vi "Toobar UI.vi"() -> ()   [LabVIEW 2016]
uses:
  System.Windows.Forms
  ToolKit/Toolbar/net/SubVIs/Pravite/ToolStrip.lvclass
  ToolKit/Toolbar/net/SubVIs/TBA_NET_Item.ctl
  <vilib>/Utility/error.llb/DialogType.ctl
  Architecture/Queue Management/ARC_Queue Create_Single.vi
  Architecture/Queue Management/ARC_Queue Remove Element.vi
  Architecture/Queue Management/ARC_Queue Insert Element.vi
  Architecture/Queue Management/ARC_Queue Destroy_Single.vi
  Architecture/Queue Management/ARC_Queue Valid.vi
panel:
  in  "ToolStrip":refnum<k24>(container)
  in  "Parameter":cluster{"Q_Local":string, "变体":variant}
  in  "TempVariable":T2 {"TBAConstant"."Item"."Stop"."DisplayStyle" items=["None", "Text", "Image", "ImageAndText"]}
  out "ToolbarClick":string
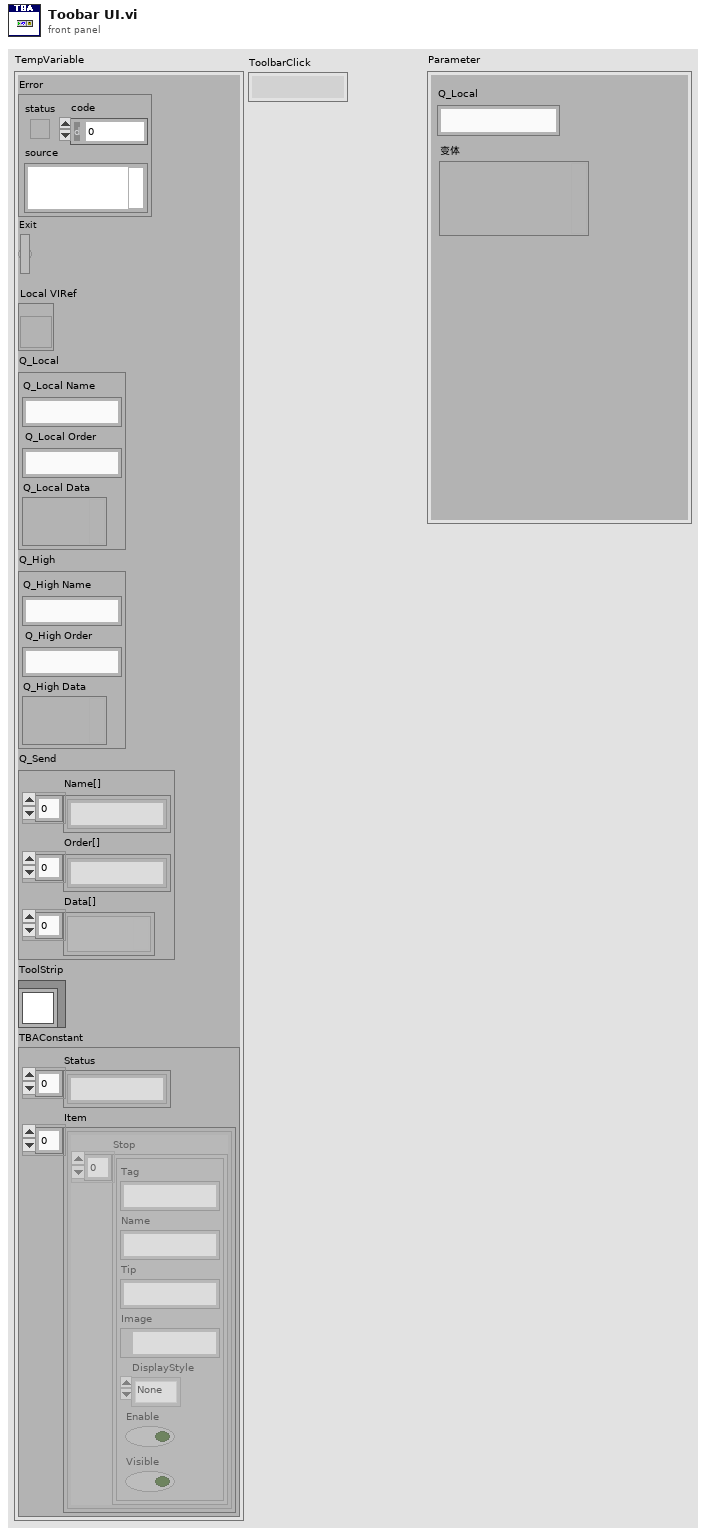
[diagram p1: front panel]
types:
  T1 = typedef "TBA_NET_Item.ctl" = cluster{"Tag":string, "Name":string, "Tip":string, "Image":path, "DisplayStyle":i32, "Enable":bool, "Visible":bool}
  T2 = cluster{"Error":errorcluster, "Exit":bool, "Local VIRef":refnum<vi>, "Q_Local":cluster{"Q_Local Name":string, "Q_Local Order":string, "Q_Local Data":variant}, "Q_High":cluster{"Q_High Name":string, "Q_High Order":string, "Q_High Data":variant}, "Q_Send":cluster{"Name[]":string[], "Order[]":string[], "Data[]":variant[]}, "ToolStrip":refnum<class "ToolStrip.lvclass">, "TBAConstant":cluster{"Status":string[], "Item":cluster{"Stop":T1[]}[]}}
  T3 = cluster{"Status":string[], "Item":cluster{"Stop":T1[]}[]}
  T4 = cluster{"Q_Local":string, "type":cluster{"Status":string[], "Item":cluster{"Stop":T1[]}[]}}
  T5 = typedef "DialogType.ctl" = u16
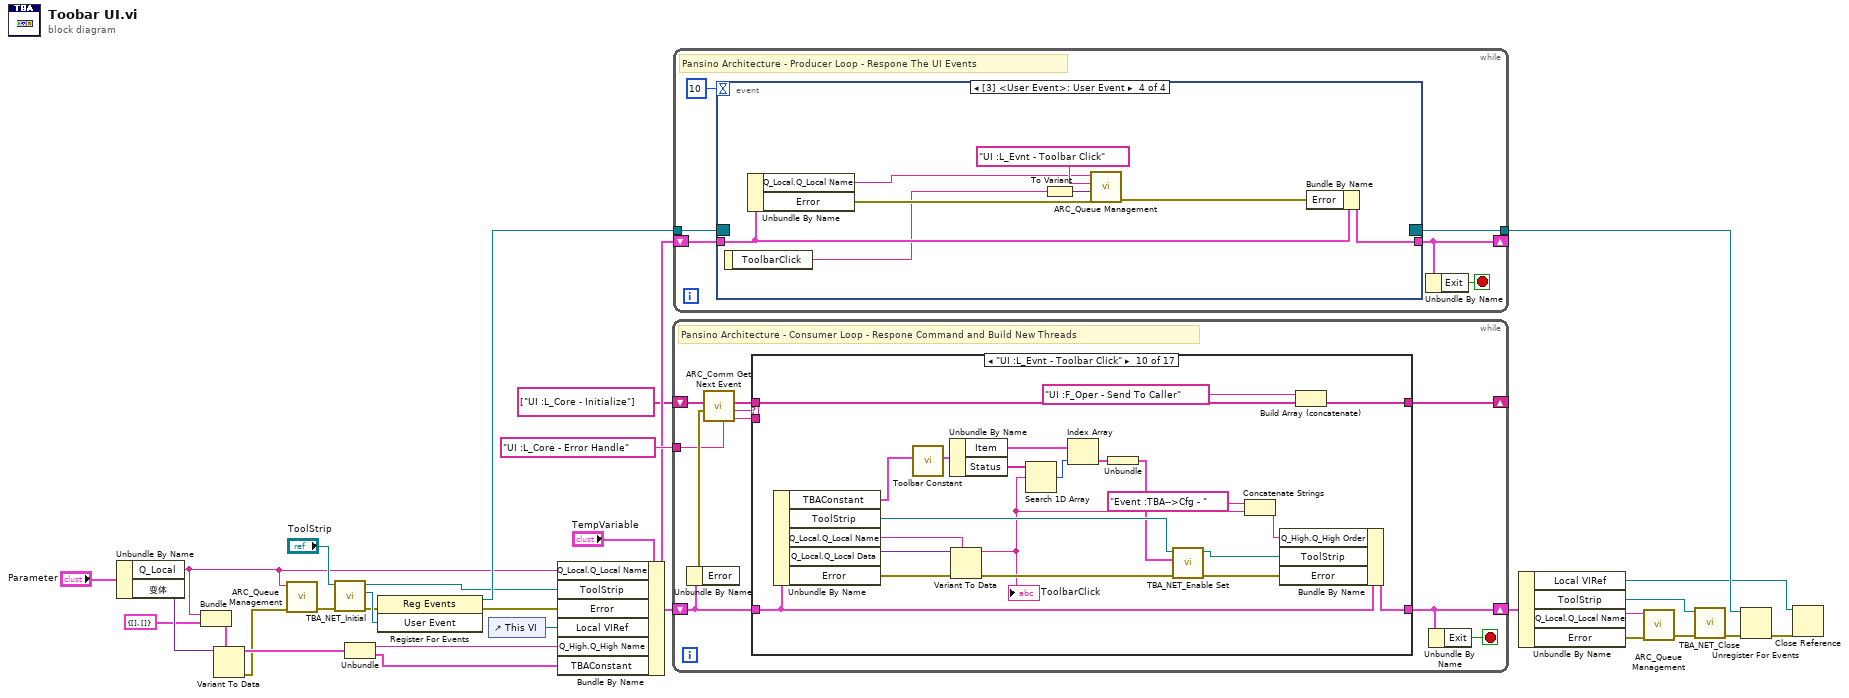
[diagram p0: block diagram]
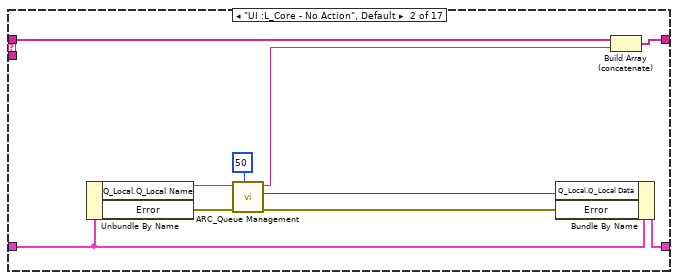
[diagram p3: hidden frame]
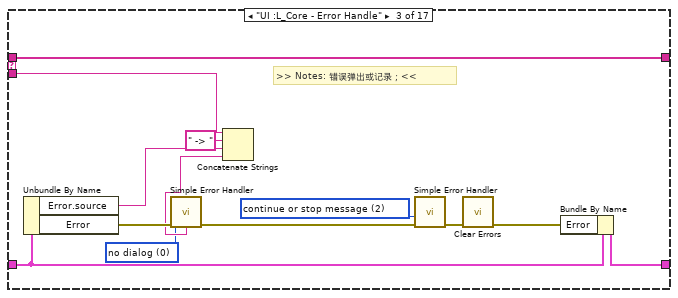
[diagram p4: hidden frame]
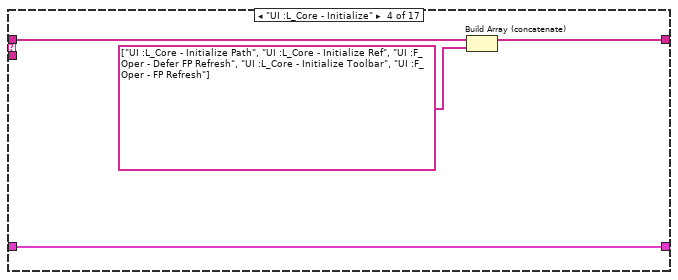
[diagram p5: hidden frame]
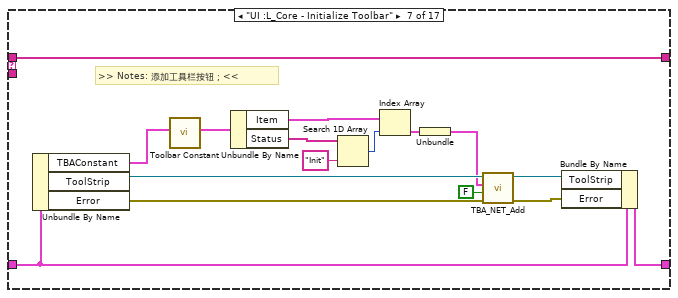
[diagram p8: hidden frame]
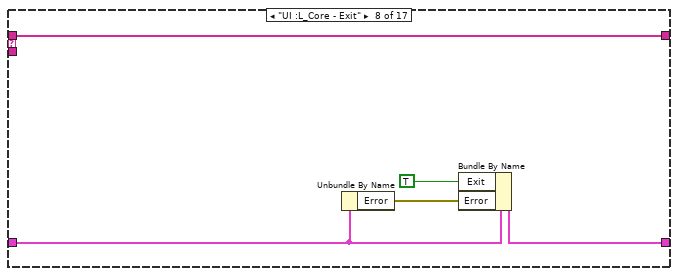
[diagram p9: hidden frame]
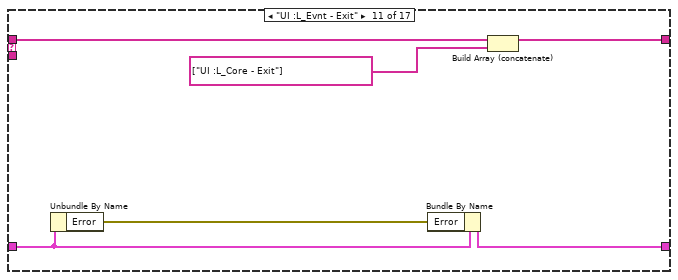
[diagram p11: hidden frame]
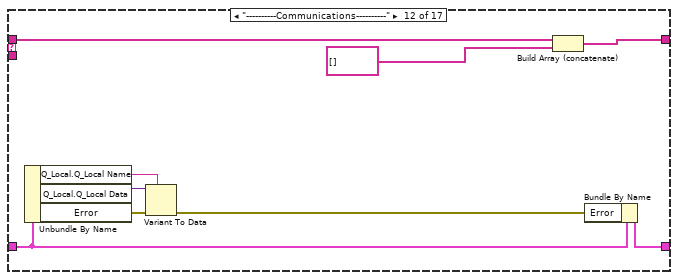
[diagram p12: hidden frame]
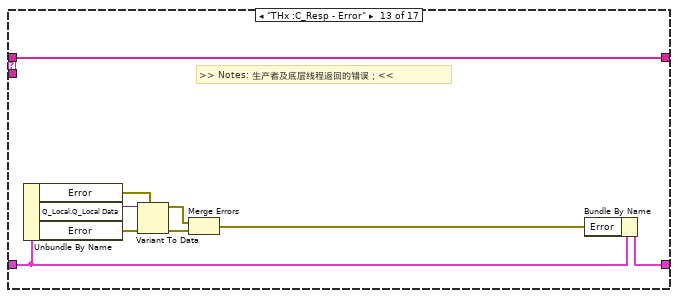
[diagram p13: hidden frame]
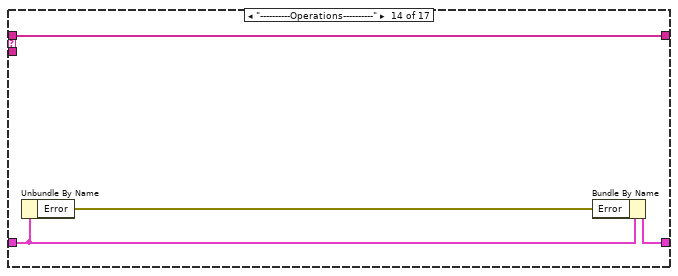
[diagram p14: hidden frame]
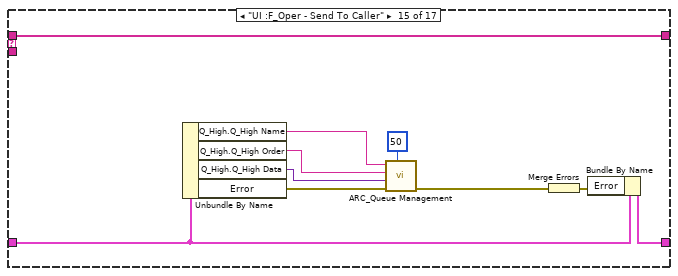
[diagram p15: hidden frame]
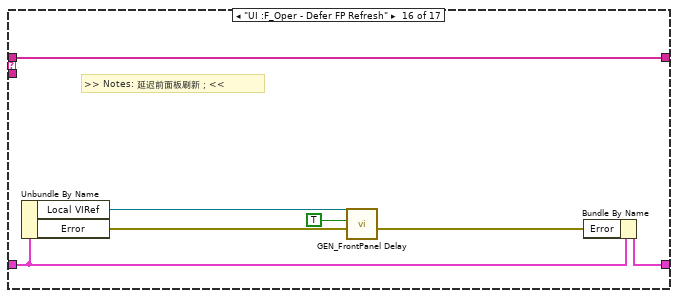
[diagram p16: hidden frame]
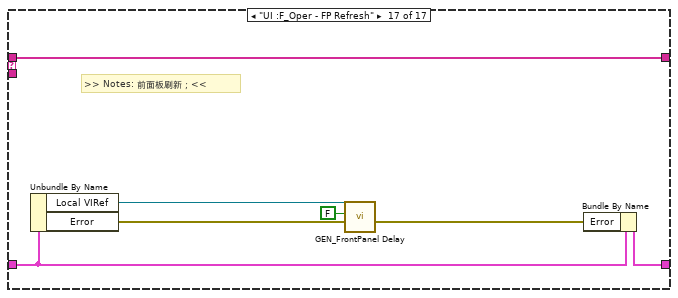
[diagram p17: hidden frame]
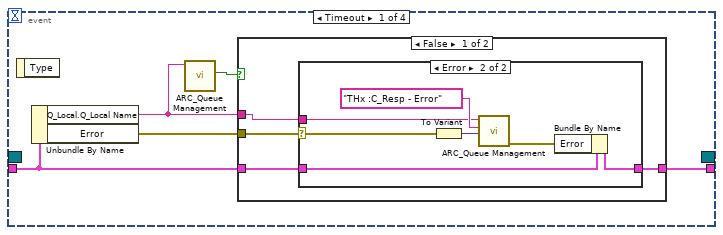
[diagram p18: hidden frame]
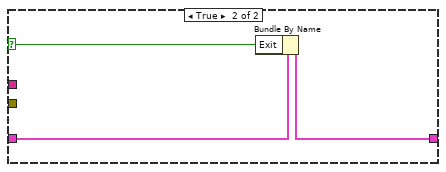
[diagram p20: hidden frame]
diagram:
  n1 = Unbundle By Name("Parameter") -> ("Q_Local"=w4:string, "变体"=w8:variant)
  n2 = Bundle("Q_Local"=w4, "type"=T3 {"Status"=[], "Item"=[]}) -> (w3:T4)  [unwired: 1 in]
  n3 = Variant To Data(type=w3, Variant=w8) -> (data=w7:T4, error out=w6:errorcluster)  [unwired: 1 in]
  n4 = call-poly "ARC_Queue Management.vi"("error in"=w6, "Queue Name"=w4) -> ("error out"=w20:errorcluster)  [unwired: 7 in, 2 out]
  n5 = call "TBA_NET_Initial.vi"("error in (no error)"=w20, "ToolStrip"="ToolStrip") -> ("error out"=w21:errorcluster, "User Event"=w22:refnum<user-event>, "ToolStrip Out"=w17:refnum<class "ToolStrip.lvclass">)  [unwired: 7 in]
  n6 = Unbundle(w7) -> ("Q_Local"=w1:string, "type"=w2:T3)
  n7 = register-events(error in=w21, w22) -> (reference out=w18:refnum<event-registration>, error out=w19:errorcluster)  [unwired: 1 in]
  n8 = control-ref of="This VI"() -> (w28:refnum<vi>)
  n9 = Bundle By Name(cluster="TempVariable", "Q_Local.Q_Local Name"=w4, "ToolStrip"=w17, "Error"=w19, "Local VIRef"=w28, "Q_High.Q_High Name"=w1, "TBAConstant"=w2) -> (w29:T2)
  n10 = while {
    shift-right: [w34] -> w24
    shift-left: w29 -> [w36]
    shift-right: [w37] -> _
    shift-left: string[] ["UI :L_Core - Initialize"] -> [w40]
    tunnel: "UI :L_Core - Error Handle" ("Error Handle") -> [w32]
    stop <- w33 stop-if-true
    # "Pansino Architecture - Consumer Loop - Respone Command and Build New Threads"
    n11 = Unbundle By Name(w36) -> ("Error"=w35:errorcluster)
    n12 = call "ARC_Comm Get Next Event.vi"("Error Handle"=w32, "error in (no error)"=w35, "event queue in"=w40) -> ("prev event"=w31:string, "next event"=w39:string, "event queue out"=w38:string[])  [unwired: 3 in]
    n13 = case shown="\"UI :L_Evnt - Toolbar Click\"" w39 {
      tunnel: w36 -> [w41 w49 w63 w68 w70 w72 w88 w91 w95 w116 w123 w130 w142 w145 w149 w162 w169]
      tunnel: w38 -> [w42 w47 w65 w69 w71 w73 w89 w94 w96 w118 w121 w133 w137 w146 w156 w163 w170]
      tunnel: [w42 w46 w65 w67 w71 w73 w89 w94 w96 w117 w120 w132 w137 w146 w156 w163 w170] -> w37
      tunnel: [w41 w48 w64 w68 w70 w72 w87 w92 w95 w115 w122 w129 w141 w144 w150 w161 w168] -> w34
      tunnel: w31 -> [_ _ w54 _ _ _ _ _ _ _ _ _ _ _ _ _ _]
      frame "----------Core Status----------" {
      }
      frame "UI :L_Core - No Action", Default {
        n14 = Unbundle By Name(w49) -> ("Q_Local.Q_Local Name"=w44:string, "Error"=w50:errorcluster)
        n15 = call-poly "ARC_Queue Management.vi"("Time out(-1)_queue out"=50, "error in (no error)"=w50, "Queue Name(unamed)"=w44) -> ("error out"=w52:errorcluster, "Data"=w51:variant, "Event"=w45:string)  [unwired: 5 in, 1 out]
        n16 = Bundle By Name(cluster=w49, "Q_Local.Q_Local Data"=w51, "Error"=w52) -> (w48:T2)
        n17 = Build Array (concatenate)(w47, w45) -> (w46:string[])
      }
      frame "UI :L_Core - Error Handle" {
        w53 = T5 0 items=["no dialog", "OK message", "continue or stop message", "OK message + warnings", "continue/stop + warnings"] ("type of dialog (OK msg:1)")
        w60 = T5 2 items=["no dialog", "OK message", "continue or stop message", "OK message + warnings", "continue/stop + warnings"] ("type of dialog (OK msg:1)")
        # ">> Notes: 错误弹出或记录；<<"
        n18 = Unbundle By Name(w63) -> ("Error.source"=w55:string, "Error"=w58:errorcluster)
        n19 = call <vilib>:"Simple Error Handler.vi"("type of dialog (OK msg:1)"=w53, "error in (no error)"=w58) -> ("error out"=w57:errorcluster, "message"=w56:string)  [unwired: 3 in, 3 out]
        n20 = Concatenate Strings(w54, " -> " ("字符串"), w55, w56) -> ()  [unwired: 1 out]
        n21 = call <vilib>:"Simple Error Handler.vi"("type of dialog (OK msg:1)"=w60, "error in (no error)"=w57) -> ("error out"=w62:errorcluster)  [unwired: 3 in, 4 out]
        n22 = call <vilib>:"Clear Errors.vi"("error in (no error)"=w62) -> ("error out"=w61:errorcluster)  [unwired: 5 in, 1 out]
        n23 = Bundle By Name(cluster=w63, "Error"=w61) -> (w64:T2)
      }
      frame "UI :L_Core - Initialize" {
        n24 = Build Array (concatenate)(w69, string[] ["UI :L_Core - Initialize Path", "UI :L_Core - Initialize Ref", "UI :F_Oper - Defer FP Refresh", "UI :L_Core - Initialize Toolbar", "UI :F_Oper - FP Refresh"] ("数组")) -> (w67:string[])
      }
      frame "UI :L_Core - Initialize Path" {
      }
      frame "UI :L_Core - Initialize Ref" {
      }
      frame "UI :L_Core - Initialize Toolbar" {
        # ">> Notes: 添加工具栏按钮；<<"
        n25 = Unbundle By Name(w88) -> ("TBAConstant"=w75:T3, "ToolStrip"=w85:refnum<class "ToolStrip.lvclass">, "Error"=w86:errorcluster)
        n26 = call "Toolbar Constant.vi"("TBA Constant in"=w75) -> ("Toolbar"=w76:T3)  [unwired: 10 in]
        n27 = Unbundle By Name(w76) -> ("Item"=w79:cluster{"Stop":T1[]}[], "Status"=w80:string[])
        n28 = Search 1D Array(1D array=w80, element="Init" ("元素")) -> (index of element=w81:i32)  [unwired: 1 in]
        n29 = Index Array(array=w79, index=w81) -> (element=w78:cluster{"Stop":T1[]})
        n30 = Unbundle(w78) -> ("Stop"=w77:T1[])
        n31 = call "TBA_NET_Add.vi"("error in (no error)"=w86, "Clear First?"=FALSE, "Item[]"=w77, "Toolbar Ref"=w85) -> ("error out"=w83:errorcluster, "ToolStrip"=w84:refnum<class "ToolStrip.lvclass">)  [unwired: 6 in]
        n32 = Bundle By Name(cluster=w88, "ToolStrip"=w84, "Error"=w83) -> (w87:T2)
      }
      frame "UI :L_Core - Exit" {
        n33 = Unbundle By Name(w91) -> ("Error"=w93:errorcluster)
        n34 = Bundle By Name(cluster=w91, "Exit"=TRUE, "Error"=w93) -> (w92:T2)
      }
      frame "----------Events----------" {
      }
      frame "UI :L_Evnt - Toolbar Click" {
        n35 = Unbundle By Name(w116) -> ("TBAConstant"=w100:T3, "ToolStrip"=w110:refnum<class "ToolStrip.lvclass">, "Q_Local.Q_Local Name"=w112:string, "Q_Local.Q_Local Data"=w113:variant, "Error"=w114:errorcluster)
        n36 = call "Toolbar Constant.vi"("TBA Constant in"=w100) -> ("Toolbar"=w102:T3)  [unwired: 10 in]
        n37 = Unbundle By Name(w102) -> ("Item"=w105:cluster{"Stop":T1[]}[], "Status"=w106:string[])
        n38 = Variant To Data(error in=w114, type=w112, Variant=w113) -> (data=w99:string, error out=w111:errorcluster)
        "ToolbarClick" <- w99
        n39 = Search 1D Array(1D array=w106, element=w99) -> (index of element=w107:i32)  [unwired: 1 in]
        n40 = Index Array(array=w105, index=w107) -> (element=w104:cluster{"Stop":T1[]})
        n41 = Unbundle(w104) -> ("Stop"=w103:T1[])
        n42 = call "TBA_NET_Enable Set.vi"("error in (no error)"=w111, "Item[]"=w103, "ToolStrip 输入"=w110) -> ("error out"=w109:errorcluster, "ToolStrip 输出"=w108:refnum<class "ToolStrip.lvclass">)  [unwired: 7 in]
        n43 = Concatenate Strings("Event :TBA-->Cfg - ", w99) -> (w97:string)
        n44 = Bundle By Name(cluster=w116, "Q_High.Q_High Order"=w97, "ToolStrip"=w108, "Error"=w109) -> (w115:T2)
        n45 = Build Array (concatenate)("UI :F_Oper - Send To Caller", w118) -> (w117:string[])
      }
      frame "UI :L_Evnt - Exit" {
        n46 = Unbundle By Name(w123) -> ("Error"=w124:errorcluster)
        n47 = Bundle By Name(cluster=w123, "Error"=w124) -> (w122:T2)
        n48 = Build Array (concatenate)(w121, string[] ["UI :L_Core - Exit"] ("数组")) -> (w120:string[])
      }
      frame "----------Communications----------" {
        n49 = Unbundle By Name(w130) -> ("Q_Local.Q_Local Name"=w125:string, "Q_Local.Q_Local Data"=w126:variant, "Error"=w128:errorcluster)
        n50 = Variant To Data(error in=w128, type=w125, Variant=w126) -> (error out=w127:errorcluster)  [unwired: 1 out]
        n51 = Build Array (concatenate)(w133, string[] [] ("数组")) -> (w132:string[])
        n52 = Bundle By Name(cluster=w130, "Error"=w127) -> (w129:T2)
      }
      frame "THx :C_Resp - Error" {
        # ">> Notes: 生产者及底层线程返回的错误；<<"
        n53 = Unbundle By Name(w142) -> ("Error"=w138:errorcluster, "Q_Local.Q_Local Data"=w139:variant, "Error"=w140:errorcluster)
        n54 = Variant To Data(error in=w140, type=w138, Variant=w139) -> (data=w136:errorcluster, error out=w135:errorcluster)
        n55 = Merge Errors(w136, w135) -> (w134:errorcluster)
        n56 = Bundle By Name(cluster=w142, "Error"=w134) -> (w141:T2)
      }
      frame "----------Operations----------" {
        n57 = Unbundle By Name(w145) -> ("Error"=w143:errorcluster)
        n58 = Bundle By Name(cluster=w145, "Error"=w143) -> (w144:T2)
      }
      frame "UI :F_Oper - Send To Caller" {
        n59 = Unbundle By Name(w149) -> ("Q_High.Q_High Name"=w151:string, "Q_High.Q_High Order"=w147:string, "Q_High.Q_High Data"=w153:variant, "Error"=w152:errorcluster)
        n60 = call-poly "ARC_Queue Management.vi"("Time out(-1)_queue in"=50, "error in (no error)"=w152, "Data"=w153, "Event"=w147, "Queue Name(unamed)"=w151) -> ("error out"=w154:errorcluster)  [unwired: 5 in, 1 out]
        n61 = Merge Errors(w154) -> (w155:errorcluster)
        n62 = Bundle By Name(cluster=w149, "Error"=w155) -> (w150:T2)
      }
      frame "UI :F_Oper - Defer FP Refresh" {
        # ">> Notes: 延迟前面板刷新；<<"
        n63 = Unbundle By Name(w162) -> ("Local VIRef"=w157:refnum<vi>, "Error"=w159:errorcluster)
        n64 = call "GEN_FrontPanel Delay.vi"("VI ref"=w157, "错误输入（无错误）"=w159, "delay？"=TRUE ("Delay?")) -> ("错误输出"=w158:errorcluster)  [unwired: 8 in]
        n65 = Bundle By Name(cluster=w162, "Error"=w158) -> (w161:T2)
      }
      frame "UI :F_Oper - FP Refresh" {
        # ">> Notes: 前面板刷新；<<"
        n66 = Unbundle By Name(w169) -> ("Local VIRef"=w164:refnum<vi>, "Error"=w166:errorcluster)
        n67 = call "GEN_FrontPanel Delay.vi"("VI ref"=w164, "错误输入（无错误）"=w166, "delay？"=FALSE ("Delay?")) -> ("错误输出"=w165:errorcluster)  [unwired: 8 in]
        n68 = Bundle By Name(cluster=w169, "Error"=w165) -> (w168:T2)
      }
    }
    n69 = Unbundle By Name(w34) -> ("Exit"=w33:bool)
  }
  n70 = while {
    shift-right: [w176] -> _
    shift-left: w29 -> [w174]
    tunnel: w18 -> [w173]
    tunnel: [w172] -> w16
    stop <- w175 stop-if-true
    # "Pansino Architecture - Producer Loop - Respone The UI Events"
    n71 = event shown="[3] <User Event>: User Event" {
      selector: w173 -> [_ _ _ _]
      dyn-events: [_ _ _ _] -> w172
      timeout: 10 -> [_ _ _ _]
      tunnel: w174 -> [w178 w201 w205 w215]
      tunnel: [w177 w200 w204 w214] -> w176
      event Timeout {
        n72 = event-data() -> ()  [unwired: 1 in, 1 out]
        n73 = Unbundle By Name(w178) -> ("Q_Local.Q_Local Name"=w180:string, "Error"=w179:errorcluster)
        n74 = call-poly "ARC_Queue Management.vi"("Queue Name(unamed)"=w180) -> ("Not Exist?"=w181:bool)  [unwired: 8 in, 2 out]
        n75 = case shown="False" w181 {
          selector: w181 -> [_ w194]
          tunnel: w178 -> [w185 w196]
          tunnel: [w183 w195] -> w177
          tunnel: w179 -> [w182 _]
          tunnel: w180 -> [w184 _]
          frame False {
            n76 = case shown="Error" w182 {
              selector: w182 -> [_ w187]
              tunnel: w185 -> [w186 w192]
              tunnel: w184 -> [_ w191]
              tunnel: [w186 w189] -> w183
              frame No Error {
              }
              frame Error {
                n77 = To Variant(anything=w187) -> (Variant=w190:variant)
                n78 = call-poly "ARC_Queue Management.vi"("Data"=w190, "Event"="THx :C_Resp - Error", "Queue Name(unamed)"=w191) -> ("error out"=w188:errorcluster)  [unwired: 7 in, 1 out]
                n79 = Bundle By Name(cluster=w192, "Error"=w188) -> (w189:T2)
              }
            }
          }
          frame True {
            n80 = Bundle By Name(cluster=w196, "Exit"=w194) -> (w195:T2)
          }
        }
      }
      event Panel Close? {
        n81 = event-data() -> ()  [unwired: 1 in, 1 out]
        n82 = Unbundle By Name(w201) -> ("Q_Local.Q_Local Name"=w197:string, "Error"=w202:errorcluster)
        n83 = call-poly "ARC_Queue Management.vi"("error in (no error)"=w202, "Event"="UI :L_Core - Exit", "Queue Name(unamed)"=w197) -> ("error out"=w199:errorcluster)  [unwired: 7 in, 1 out]
        n84 = Bundle By Name(cluster=w201, "Error"=w199) -> (w200:T2)
        n85 = event-data("Discard?"=TRUE ("放弃？")) -> ()  [unwired: 1 in, 1 out]
      }
      event Mouse Enter {
        n86 = event-data() -> ()  [unwired: 1 in, 4 out]
        n87 = Unbundle By Name(w205) -> ("Error"=w207:errorcluster)
        n88 = control-ref of="本VI"() -> (w209:refnum<vi>)
        n89 = property class="VI"(reference=w209, error in=w207, "Front Panel.IsFrontmost"=TRUE ("前面板窗口:在最前")) -> (error out=w206:errorcluster)  [unwired: 1 out]
        n90 = Bundle By Name(cluster=w205, "Error"=w206) -> (w204:T2)
      }
      event User Event {
        n91 = event-data() -> ("ToolbarClick"=w210:string)  [unwired: 1 in]
        n92 = Unbundle By Name(w215) -> ("Q_Local.Q_Local Name"=w212:string, "Error"=w216:errorcluster)
        n93 = To Variant(anything=w210) -> (Variant=w211:variant)
        n94 = call-poly "ARC_Queue Management.vi"("error in (no error)"=w216, "Data"=w211, "Event"="UI :L_Evnt - Toolbar Click", "Queue Name(unamed)"=w212) -> ("error out"=w213:errorcluster)  [unwired: 6 in, 1 out]
        n95 = Bundle By Name(cluster=w215, "Error"=w213) -> (w214:T2)
      }
    }
    n96 = Unbundle By Name(w176) -> ("Exit"=w175:bool)
  }
  n97 = Unbundle By Name(w24) -> ("Local VIRef"=w10:refnum<vi>, "ToolStrip"=w15:refnum<class "ToolStrip.lvclass">, "Q_Local.Q_Local Name"=w27:string, "Error"=w25:errorcluster)
  n98 = call-poly "ARC_Queue Management.vi"("error in (no error)"=w25, "Queue Name(unamed)"=w27) -> ("error out"=w14:errorcluster)  [unwired: 7 in, 2 out]
  n99 = call "TBA_NET_Close.vi"("error in (no error)"=w14, "ToolStrip 输入"=w15) -> ("error out"=w13:errorcluster)  [unwired: 9 in]
  n100 = Unregister For Events(event registration refnum=w16, error in=w13) -> (error out=w11:errorcluster)
  n101 = Close Reference(reference=w10, error in (no error)=w11) -> ()  [unwired: 1 out]
